vi "Find Workspace.vi"(6 "Pickup_Test_Number":dbl, 7 "Database Entry in":refnum<class "Database Entry.lvclass">, 8 "error in (no error)":errorcluster, 9 "Assembly Type":string, 10 "Control In":T2={"I-O.lvclass"=refnum, "Gantry"=refnum, "Dispenser"="COM1"}, 11 "Component.lvclass":refnum<class "Component Tray.lvclass">) -> (0 "error out":errorcluster, 1 "Workspace":T1, 2 "Control Out":T2={"I-O.lvclass"=refnum, "Gantry"=refnum, "Dispenser"="COM1"}, 3 "Workspace Out":refnum<class "Component Tray.lvclass">, 5 "Database Entry out":refnum<class "Database Entry.lvclass">)   [LabVIEW 2021, in "Component Tray.lvclass"]
uses:
  Component Tray.lvclass
  Controller/Controllers.ctl
  Controller/I-O/I-O.lvclass
  C:/Program Files (x86)/Aerotech/A3200/LabVIEW/2010/Bin/Aerotech.A3200.dll
  Program Files (x86)/Aerotech/A3200/LabVIEW/2010/Bin/Aerotech.A3200.dll
  Workspace.ctl
  C:/Users/HEP/Documents/GitHub/Gantry/UCSB-Gantry-HEP-main/Classes/Workspace/Fixture.lvclass
  Assembly/Database Entry/Database Entry.lvclass
  Fixture.lvclass/Fixture.ctl
  Component Tray.lvclass/Component Tray.ctl
  Read Fixture ID.vi
  Read Position.vi
  Fixture.lvclass
  Controller/Controller.lvclass
panel:
  out "XYZTheta":dbl[](array[numeric]) format="%#.6g"
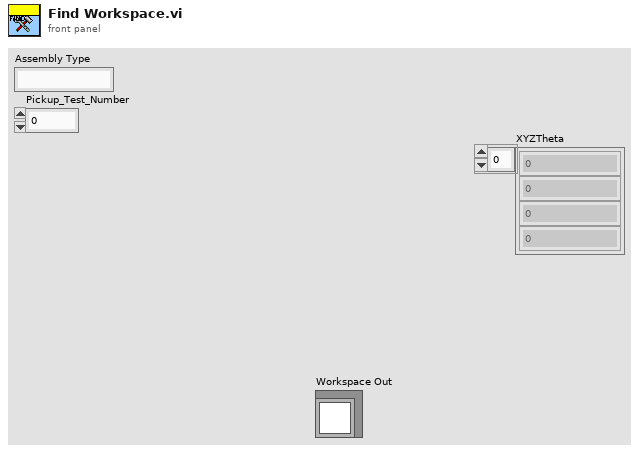
[diagram p1: front panel]
types:
  T1 = typedef "Fixture.lvclass/Workspace.ctl" = cluster{"XYZTheta":dbl[], "Workspace Valve":i32, "Workspace Sensor":i32, "Tray Number":i32, "Position":i32, "Assembly Type":string, "Numeric":dbl, "First Pos":i32}
  T2 = typedef "Controller.lvclass/Controllers.ctl" = cluster{"I-O.lvclass":refnum<class "I-O.lvclass">, "Gantry":refnum<k24>, "Dispenser":refnum<visa-resource-name>}
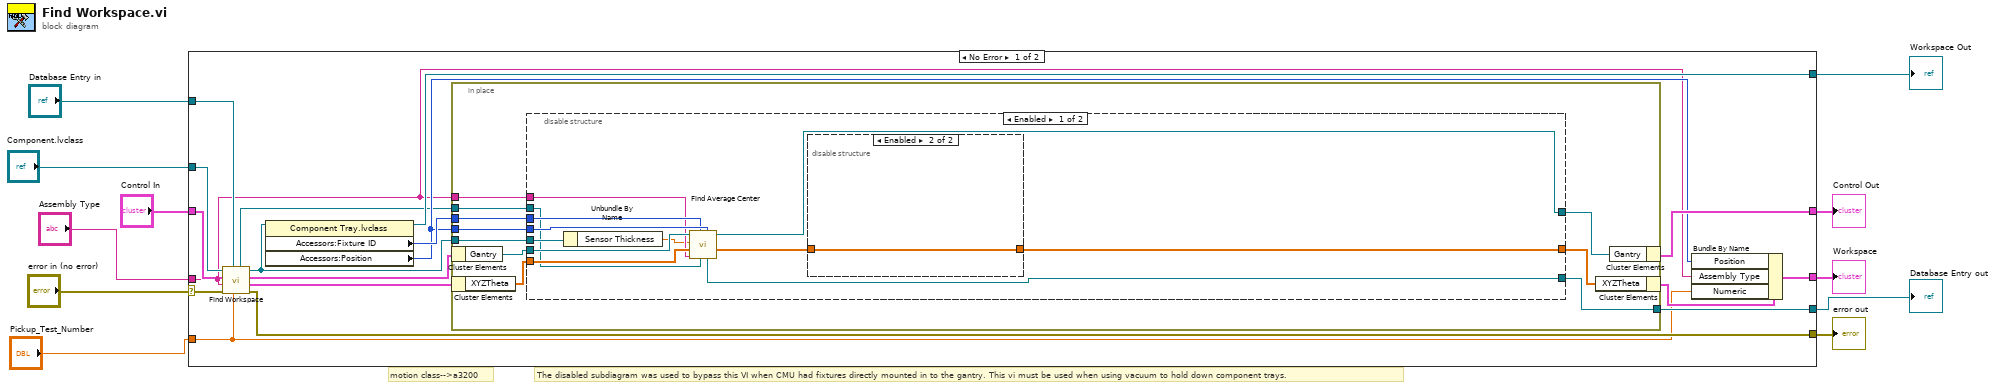
[diagram p0: block diagram]
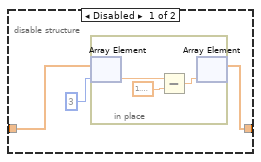
[diagram p2: hidden frame]
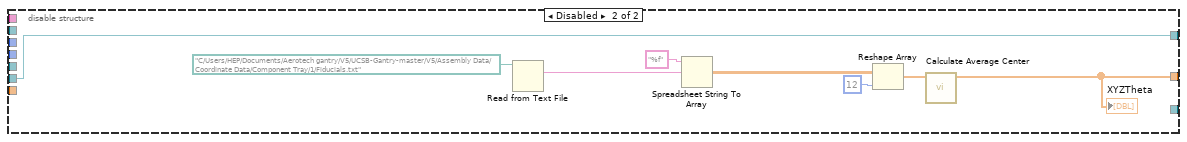
[diagram p3: hidden frame]
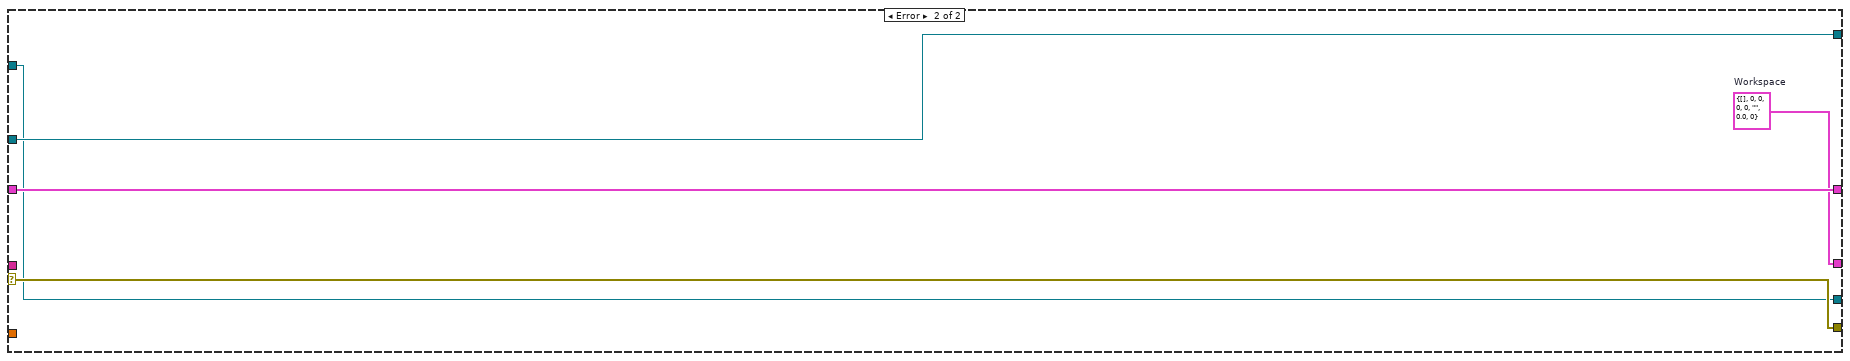
[diagram p4: hidden frame]
diagram:
  # "The disabled subdiagram was used to bypass this VI when CMU had fixtures directly mounted in to the gantry. This vi must be used when using vacuum to hold down component trays."
  # "motion class-->a3200"
  n1 = case shown="No Error" "error in (no error)" {
    selector: "error in (no error)" -> [w27 w71]
    tunnel: [w23 w70] -> w11
    tunnel: [w29 w71] -> w10
    tunnel: [w17 w69] -> w9
    tunnel: "Control In" -> [w26 w70]
    tunnel: [w21 w68] -> w6
    tunnel: "Component.lvclass" -> [w25 w68]
    tunnel: "Assembly Type" -> [w13 _]
    tunnel: "Database Entry in" -> [w15 w67]
    tunnel: [w19 w67] -> w2
    tunnel: "Pickup_Test_Number" -> [w12 _]
    frame No Error {
      n2 = call-parent "Find Workspace.vi"("Pickup_Test_Number"=w12, "Database Entry in"=w15, "Error In"=w27, "Assembly Type"=w13, "Control In"=w26, "Workspace In"=w25) -> ("Error Out"=w29:errorcluster, 1:"Workspace Out"=w28:T1, "Control Out"=w24:T2, 3:"Workspace Out"=w20:refnum<class "Component Tray.lvclass">, "Database Entry out"=w14:refnum<class "Database Entry.lvclass">)  [unwired: 1 in]
      n3 = property class="Component Tray.lvclass"(reference=w20) -> (reference out=w21:refnum<class "Component Tray.lvclass">, "Accessors:Fixture ID"=w22:i32, "Accessors:Position"=w16:i32)  [unwired: 1 in, 1 out]
      n4 = in-place {
        in-place-border: w22 -> [w38]
        in-place-border: w16 -> [w39]
        in-place-border: w13 -> [w33]
        in-place-border: w20 -> [w32]
        in-place-border: w14 -> [w31]
        in-place-border: [w30] -> w19
        n5 = in-place-cluster #1(w24) -> ("Gantry"=w37:refnum<k24>)
        n6 = in-place-cluster #2(w28) -> ("XYZTheta"=w36:dbl[])
        n7 = disable-structure shown="Enabled" {
          disable-tunnel: w39 -> [w48 _]
          disable-tunnel: w38 -> [w47 _]
          disable-tunnel: w37 -> [w51 w59]
          disable-tunnel: w36 -> [w50 _]
          disable-tunnel: [w45 w60] -> w35
          disable-tunnel: [w49 w59] -> w34
          disable-tunnel: w33 -> [w44 _]
          disable-tunnel: w32 -> [w43 _]
          disable-tunnel: w31 -> [w41 _]
          disable-tunnel: [w40 _] -> w30
          frame Enabled {
            n8 = Unbundle By Name(w43) -> ("Sensor Thickness"=w42:dbl)
            n9 = call "Find Average Center.vi"("Position"=w48, "Database Entry in"=w41, "Tray Number"=w47, "Assembly Type"=w44, "XYZTheta"=w50, "Sensor Thickness"=w42, "Gantry In"=w51) -> ("XYZTheta"=w46:dbl[], "Gantry Out"=w49:refnum<k24>, "Database Entry out"=w40:refnum<class "Database Entry.lvclass">)  [unwired: 2 in]
            n10 = disable-structure shown="Enabled" {
              disable-tunnel: w46 -> [w54 w58]
              disable-tunnel: [w52 w58] -> w45
              frame Disabled {
                n11 = in-place {
                  n12 = in-place-array #3(w54, 3) -> (w57:dbl)
                  n13 = Subtract(x=w57, y=1.5707963267948966) -> (x-y=w55:dbl)
                  n14 = in-place-array #3(w55) -> (w52:dbl[])  [unwired: 1 out]
                }
              }
              frame Enabled {
              }
            }
          }
          frame Disabled {
            n15 = Read from Text File(file (use dialog)=path "C:/Users/HEP/Documents/Aerotech gantry/V5/UCSB-Gantry-master/V5/Assembly Data/Coordinate Data/Component Tray/1/Fiducials.txt") -> (text=w64:string)  [unwired: 3 in, 3 out]
            n16 = Spreadsheet String To Array(format string="%f", spreadsheet string=w64) -> (array=w63:dbl[][])  [unwired: 2 in]
            n17 = Reshape Array(w63, 12 ("dimension size")) -> (w61:dbl[])
            n18 = call "Calculate Average Center.vi"("Gantry Fiducials"=w61) -> ("XYZTheta"=w60:dbl[])  [unwired: 8 in, 2 out]
            "XYZTheta" <- w60
          }
        }
        n19 = in-place-cluster #2("XYZTheta"=w35) -> (w18:T1)
        n20 = in-place-cluster #1("Gantry"=w34) -> (w23:T2)
      }
      n21 = Bundle By Name(cluster=w18, "Position"=w16, "Assembly Type"=w13, "Numeric"=w12) -> (w17:T1)
    }
    frame Error {
      w69 = T1 {"XYZTheta"=[], "Workspace Valve"=0, "Workspace Sensor"=0, "Tray Number"=0, "Position"=0, "Assembly Type"="", "Numeric"=0.0, "First Pos"=0}  # Workspace
    }
  }
  "error out" <- w10
  "Control Out" <- w11
  "Workspace" <- w9
  "Workspace Out" <- w6
  "Database Entry out" <- w2
